vi "Polymorphic Gain and Phase.vi"   [LabVIEW 2016]
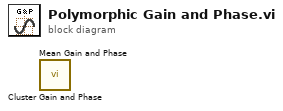
[diagram p0: block diagram]
diagram:
  n1 = call "Cluster Gain and Phase.vi"() -> ()  [unwired: 2 in, 1 out]
  n2 = call "Mean Gain and Phase.vi"() -> ()  [unwired: 2 in, 1 out]
